vi "Selects number of cores.vi"(11 "Logical cores":T1(ring)) -> (3 "Number of logical cores to use":i32)   [LabVIEW 2013, in "KLB.lvlib"]
doc: "Outputs number of CPU logical cores to use based on enum input\n\nEnum input\n\nCPU 25%\nCPU 50%\nCPU 75%\nCPU All but 1\n1\n4\n8\n16\n\nOutput\nCalculated number of CPUs to use based on input"
uses:
  KLB.lvlib
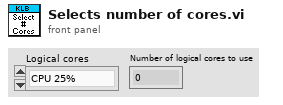
[diagram p1: front panel]
types:
  T1 = enum16{"CPU 25%", "CPU 50%", "CPU 75%", "CPU All but 1", "1", "4", "8", "16"}
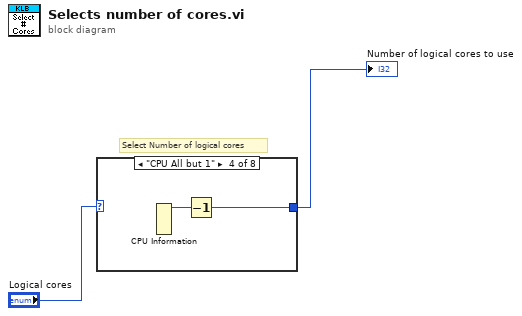
[diagram p0: block diagram]
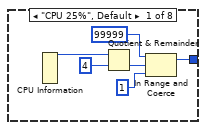
[diagram p2: hidden frame]
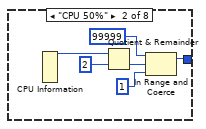
[diagram p3: hidden frame]
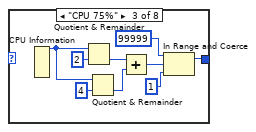
[diagram p4: hidden frame]
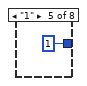
[diagram p5: hidden frame]
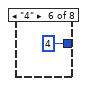
[diagram p6: hidden frame]
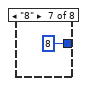
[diagram p7: hidden frame]
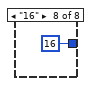
[diagram p8: hidden frame]
diagram:
  # "Select Number of logical cores"
  n1 = case shown="\"CPU All but 1\"" "Logical cores" {
    tunnel: [w4 w10 w20 w24 1 ("lower limit") 4 ("lower limit") 8 ("lower limit") 16 ("lower limit")] -> w1
    frame "CPU 25%", Default {
      n2 = CPU Information() -> (4:w5:i32)  [unwired: 3 out]
      n3 = Quotient & Remainder(x=w5, y=4) -> (floor(x/y)=w7:i32)  [unwired: 1 out]
      n4 = In Range and Coerce(upper limit=99999, x=w7, lower limit=1) -> (coerced(x)=w4:i32)  [unwired: 1 out]
    }
    frame "CPU 50%" {
      n5 = CPU Information() -> (4:w11:i32)  [unwired: 3 out]
      n6 = Quotient & Remainder(x=w11, y=2) -> (floor(x/y)=w13:i32)  [unwired: 1 out]
      n7 = In Range and Coerce(upper limit=99999, x=w13, lower limit=1) -> (coerced(x)=w10:i32)  [unwired: 1 out]
    }
    frame "CPU 75%" {
      n8 = CPU Information() -> (4:w21:i32)  [unwired: 3 out]
      n9 = Quotient & Remainder(x=w21, y=2) -> (floor(x/y)=w19:i32)  [unwired: 1 out]
      n10 = Quotient & Remainder(x=w21, y=4) -> (floor(x/y)=w18:i32)  [unwired: 1 out]
      n11 = Add(x=w19, y=w18) -> (x+y=w17:i32)
      n12 = In Range and Coerce(upper limit=99999, x=w17, lower limit=1) -> (coerced(x)=w20:i32)  [unwired: 1 out]
    }
    frame "CPU All but 1" {
      n13 = CPU Information() -> (4:w25:i32)  [unwired: 3 out]
      n14 = Decrement(x=w25) -> (x-1=w24:i32)
    }
    frame "1" {
    }
    frame "4" {
    }
    frame "8" {
    }
    frame "16" {
    }
  }
  "Number of logical cores to use" <- w1
